vi "Calculate Height for #Rocks.vi"(0 "Calculate Height for #Rocks":u64=2022, 1 "Tower Heights":map{i32, u64}(c390), 2 "Sequence Analysis":T1) -> (3 "Tower Height":u64)   [LabVIEW 2020, in "AoC 2022.lvlib"]
uses:
  AoC 2022.lvlib
  Sequence Analysis.ctl
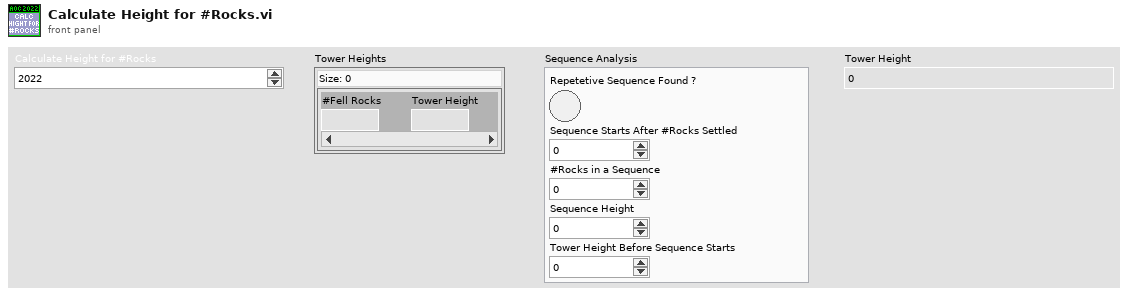
[diagram p1: front panel]
types:
  T1 = typedef "AoC 2022.lvlib/Sequence Analysis.ctl" = cluster{"Repetetive Sequence Found ?":bool, "Sequence Starts After #Rocks Settled":i32, "#Rocks in a Sequence":i32, "Sequence Height":u64, "Tower Height Before Sequence Starts":u64}
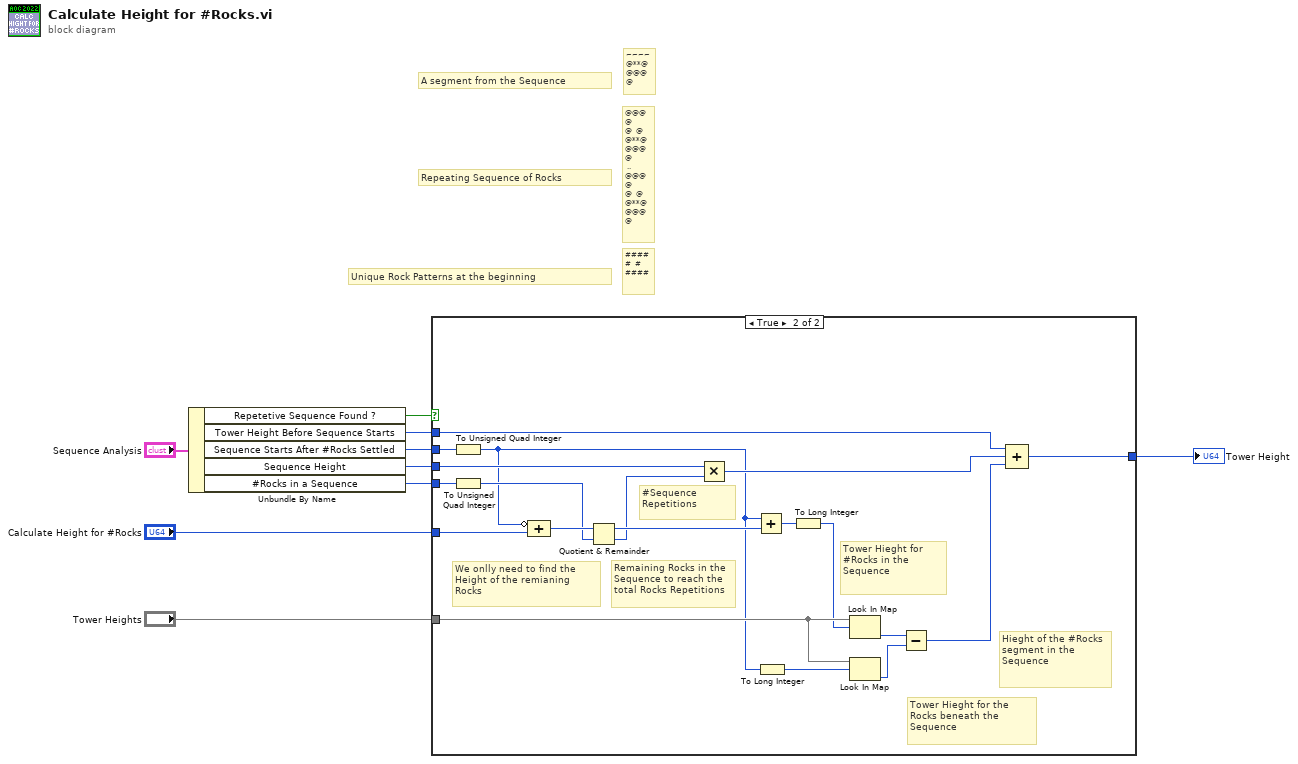
[diagram p0: block diagram]
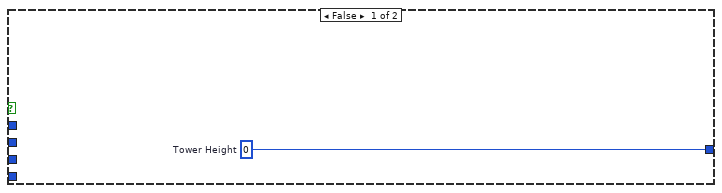
[diagram p2: hidden frame]
diagram:
  # "A segment from the Sequence"
  # "Repeating Sequence of Rocks"
  # "Unique Rock Patterns at the beginning"
  # "~~~~\n@**@\n@@@@"
  # "@@@@\n@  @\n@**@\n@@@@\n ..\n@@@@\n@  @\n@**@\n@@@@"
  # "####\n#  #\n####"
  n1 = Unbundle By Name("Sequence Analysis") -> ("Repetetive Sequence Found ?"=w7:bool, "Tower Height Before Sequence Starts"=w6:u64, "Sequence Starts After #Rocks Settled"=w5:i32, "Sequence Height"=w4:u64, "#Rocks in a Sequence"=w3:i32)
  n2 = case shown="True" w7 {
    tunnel: "Tower Heights" -> [_ w21]
    tunnel: w6 -> [_ w26]
    tunnel: w5 -> [_ w14]
    tunnel: w4 -> [_ w27]
    tunnel: w3 -> [_ w28]
    tunnel: [w10 w25] -> w2
    tunnel: "Calculate Height for #Rocks" -> [_ w29]
    frame False {
      w10 = u64 0  # Tower Height
    }
    frame True {
      # "Hieght of the #Rocks segment in the Sequence"
      # "Tower Hieght for #Rocks in the Sequence"
      # "Tower Hieght for the Rocks beneath the Sequence"
      # "Remaining Rocks in the Sequence to reach the total Rocks Repetitions"
      # "#Sequence Repetitions"
      # "We onlly need to find the Height of the remianing Rocks"
      n3 = To Unsigned Quad Integer(1:w14) -> (0:w13:u64)
      n4 = To Unsigned Quad Integer(1:w28) -> (0:w16:u64)
      n5 = Compound Arithmetic op=ADD(invert w13, w29) -> (w17:u64)
      n6 = Quotient & Remainder(x=w17, y=w16) -> (x-y*floor(x/y)=w24:u64, floor(x/y)=w15:u64)
      n7 = Multiply(x=w27, y=w15) -> (x*y=w22:u64)
      n8 = Add(x=w13, y=w24) -> (x+y=w23:u64)
      n9 = To Long Integer(number=w13) -> (32bit integer=w11:i32)
      n10 = To Long Integer(number=w23) -> (32bit integer=w12:i32)
      n11 = Look In Map(map=w21, key=w12) -> (value=w20:u64)  [unwired: 1 in, 1 out]
      n12 = Look In Map(map=w21, key=w11) -> (value=w19:u64)  [unwired: 1 in, 1 out]
      n13 = Subtract(x=w20, y=w19) -> (x-y=w18:u64)
      n14 = Compound Arithmetic op=ADD(w26, w22, w18) -> (w25:u64)
    }
  }
  "Tower Height" <- w2
